vi "MC tdms path to scan data and info path.vi"(11 "TDMS path":path) -> (2 "appended path":path, 3 "Path":path)   [LabVIEW 2020]
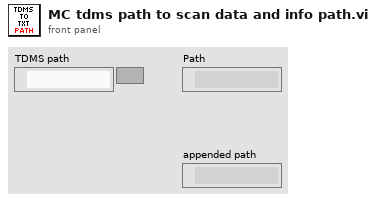
[diagram p1: front panel]
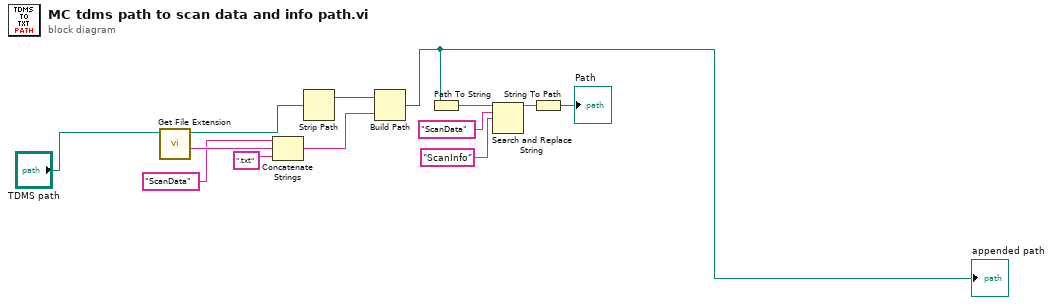
[diagram p0: block diagram]
diagram:
  n1 = call <vilib>:"Get File Extension.vi"("file"="TDMS path") -> ("filename without extension"=w6:string, "dup file"=w3:path)  [unwired: 6 in, 3 out]
  n2 = Concatenate Strings("ScanData" ("string"), w6, ".txt" ("string")) -> (w4:string)
  n3 = Strip Path(path=w3) -> (stripped path=w2:path)  [unwired: 1 out]
  n4 = Build Path(base path=w2, name or relative path=w4) -> (appended path=w12:path)
  "appended path" <- w12
  n5 = Path To String(path=w12) -> (string=w8:string)
  n6 = Search and Replace String(input string=w8, search string="ScanData", replace string="ScanInfo" ("replace string (\"\")")) -> (result string=w11:string)  [unwired: 5 in, 3 out]
  n7 = String To Path(string=w11) -> (path=→"Path":path)
